vi "Matrix_target.vi"() -> ()   [LabVIEW 2018]
uses:
  <vilib>/Platform/TimedLoop/XDataNode/timing_clust.ctl
  <vilib>/Platform/TimedLoop/XDataNode/nitl_modes.ctl
  <vilib>/Platform/TimedLoop/XDataNode/wakeup.ctl
  <vilib>/rvi/Emulation/niFpgaGetClockAttributes.vi
  <vilib>/rvi/Emulation/niFpgaSctlEmulationGetInTimedLoop.vi
  <vilib>/rvi/Emulation/niFpgaEmulationReportErrorSimple.vi
  <vilib>/rvi/Emulation/niFpgaCriticalErrorInLSC.vi
  <vilib>/rvi/eio/common/nirviEmuTemplateMethod_errors.vi
  <vilib>/rvi/Emulation/niFpgaProcessEmulError.vi
  <vilib>/Platform/TimedLoop/XDataNode/XDataNode.xnode
  <vilib>/eio/EIONode/EIONode.xnode
  <vilib>/Platform/TimedLoop/XDataNode/XDNodeRunTimeDep.lvlib
panel:
  in  "54":i16=53
  in  "36":i16=35
  in  "18":i16=17
  in  "72":i16=53
  in  "71":i16=53
  in  "17":i16=17
  in  "35":i16=35
  in  "53":i16=53
  in  "0_WE divider":i32=10
  in  "10_Rise/Fall divider":i32=3
  in  "75_Stop":i16=57
  out "Data_Array":bool[](array[boolean])
  in  "Send_Request":bool
  in  "DataLow":u64
  out "ACK":bool[](array[boolean])
  in  "/Reset_Bar":bool
  out "Sclk":bool
  in  "DataUp":u64
  in  "100_Sclk_divider":i32=25
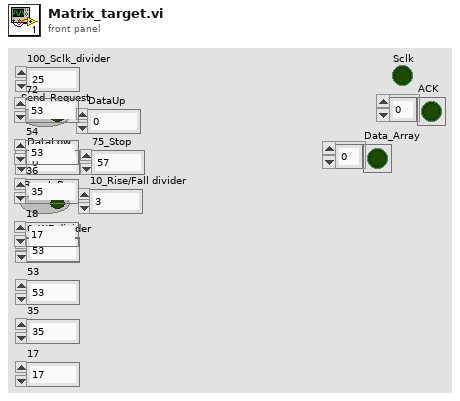
[diagram p1: front panel]
types:
  T1 = typedef "XDNodeRunTimeDep.lvlib/timing_clust.ctl" = cluster{"Expected End [f-1]":u64, "Actual End [f-1]":u64, "Finished Late? [f-1]":bool, "Expected End [i-1]":u64, "Actual End [i-1]":u64, "Finished Late? [i-1]":bool, "Expected Start [i]":u64, "Actual Start [i]":u64, "Expected Start [f]":u64, "Actual Start [f]":u64, "Source Name":string, "Structure Name":string, "Period":i64, "Deadline":i64, "Offset":i64, "Start":i64, "Priority":i32, "Timeout":i32, "Mode":T2, "Wakeup Reason":T3, "Error":errorcluster, "Source Type":string, "Secondary Source Type":string, "Global End Time":u64, "Global Start Time":u64, "Frame Duration":u64, "Iteration Duration":u64, "Assigned CPU":i32, "I/O Scan Engine Mode":u32}
  T2 = typedef "XDNodeRunTimeDep.lvlib/nitl_modes.ctl" = enum32{"No Change", "Process missed periods, maintain original phase", "Discard missed periods, maintain original phase", "Process missed periods, ignore original phase", "Discard missed periods, ignore original phase"}
  T3 = typedef "XDNodeRunTimeDep.lvlib/wakeup.ctl" = enum32{"Normal", "Aborted", "Asynchronous wakeup", "Timing source error", "Timed loop error", "Timeout"}
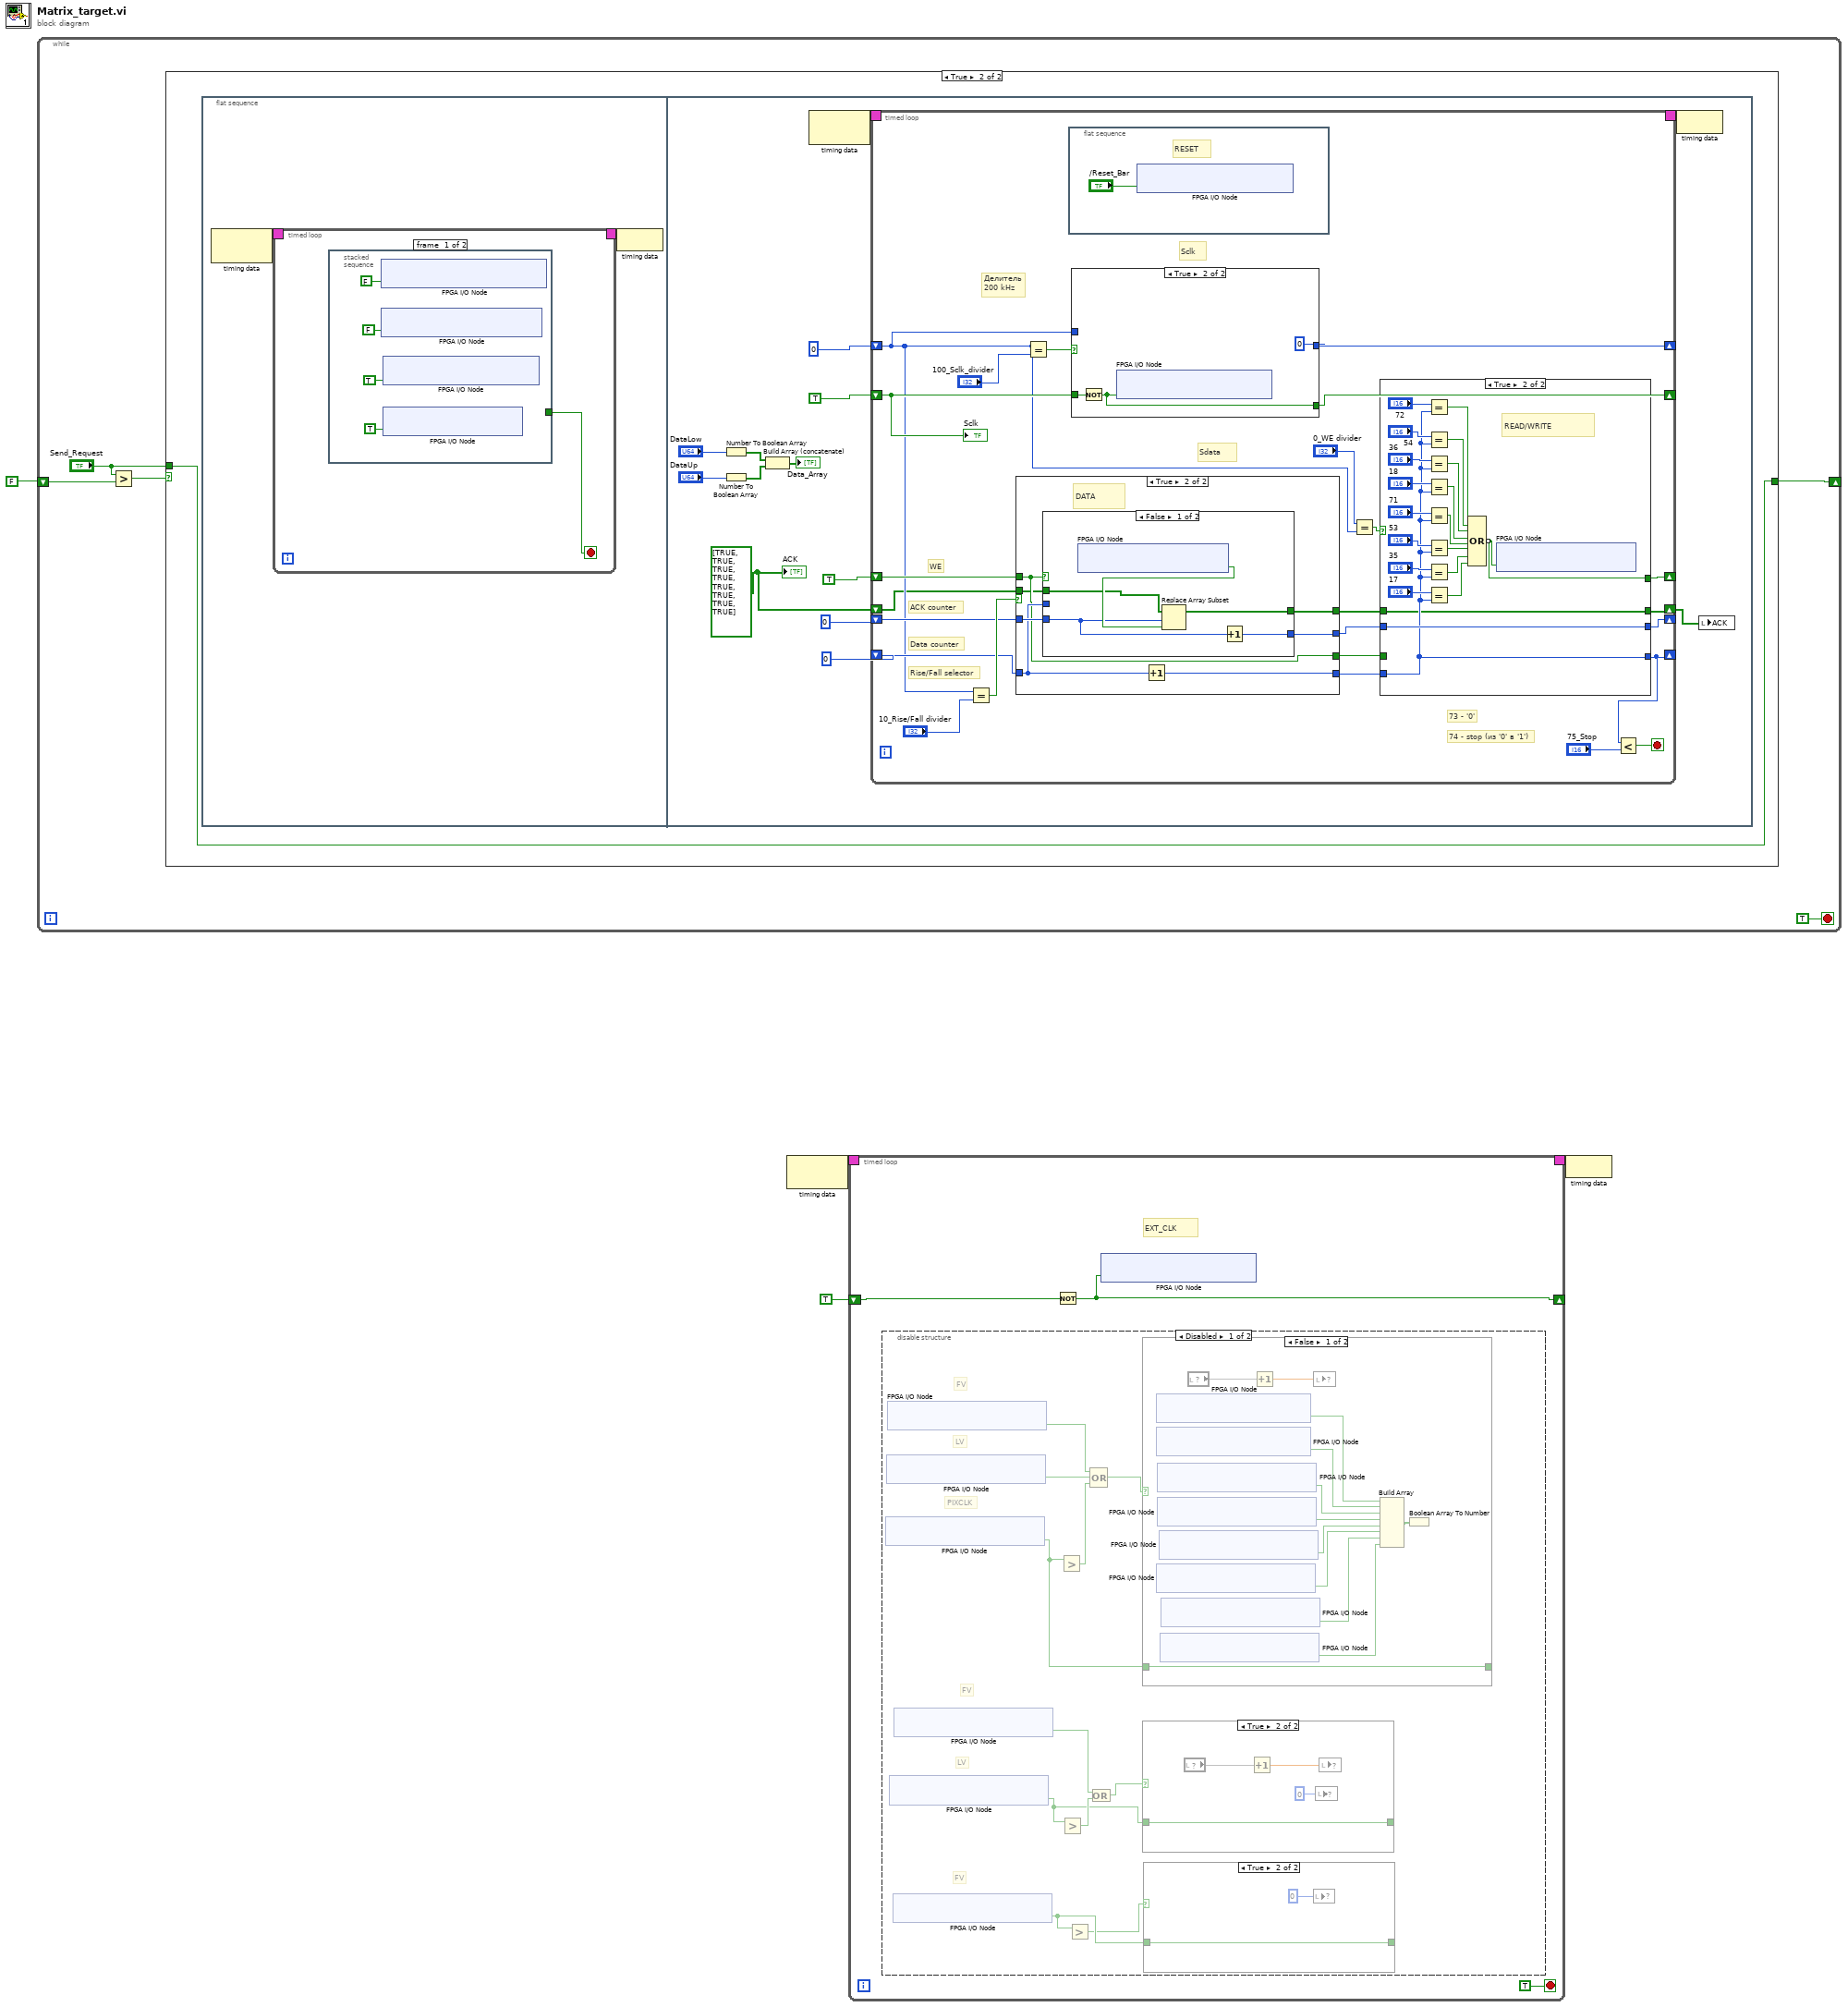
[diagram p0: block diagram]
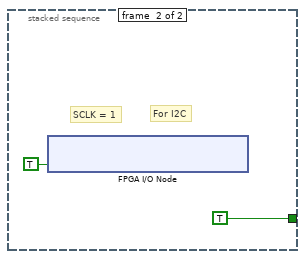
[diagram p7: hidden frame]
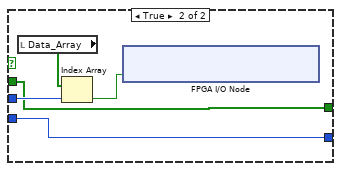
[diagram p10: hidden frame]
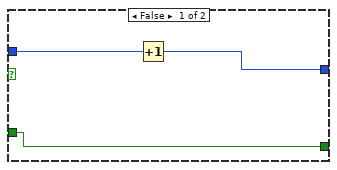
[diagram p11: hidden frame]
diagram:
  n1 = while {
    shift-right: [w8] -> _
    shift-left: FALSE ("Send_Request") -> [w7]
    stop <- TRUE stop-if-true
    n2 = Greater?(x="Send_Request", y=w7) -> (0:w6:bool)
    n3 = case shown="True" w6 {
      tunnel: "Send_Request" -> [w10 w11]
      tunnel: [w10 w11] -> w8
      frame False {
      }
      frame True {
        n4 = flat-sequence {
          frame #0 {
            n5 = node-c288() -> (w13:T1)  [unwired: 1 in]
            n6 = timed-loop {
              timing: w13 -> [_]
              timing-out: [_] -> w12
              stop <- w14 stop-if-true
              n7 = stacked-sequence {
                tunnel: [_ TRUE] -> w14
                frame #0 {
                  n8 = xnode "FPGA I/O Node"("IO Module\\DDCA_DIO16-23_WE"=FALSE ("IO Module\\DDCA_DIO16-23_WE")) -> ()  [unwired: 1 in, 1 out]
                  n9 = xnode "FPGA I/O Node"("IO Module\\DDCA_DIO8-15_WE"=FALSE ("IO Module\\DDCA_DIO8-15_WE")) -> ()  [unwired: 1 in, 1 out]
                  n10 = xnode "FPGA I/O Node"("IO Module\\DDCA_DIO0-7_WE"=TRUE ("IO Module\\DDCA_DIO0-7_WE")) -> ()  [unwired: 1 in, 1 out]
                  n11 = xnode "FPGA I/O Node"("IO Module\\DDCA_PFI_WE"=TRUE ("IO Module\\DDCA_DIO0-7_WE")) -> ()  [unwired: 1 in, 1 out]
                }
                frame #1 {
                  # "For I2C"
                  # "SCLK = 1"
                  n12 = xnode "FPGA I/O Node"("IO Module\\DDCA_DIO6_Write"=TRUE ("IO Module\\DDCA_DIO6_Write")) -> ()  [unwired: 1 in, 1 out]
                }
              }
            }
            n13 = node-c288(w12) -> ()
          }
          frame #1 {
            w25 = bool[] [TRUE, TRUE, TRUE, TRUE, TRUE, TRUE, TRUE, TRUE] ("ACK")
            n14 = Number To Boolean Array(number="DataLow") -> (Boolean array=w32:bool[])
            n15 = Number To Boolean Array(number="DataUp") -> (Boolean array=w31:bool[])
            n16 = Build Array (concatenate)(w32, w31) -> (→"Data_Array":bool[])
            n17 = node-c288() -> (w38:T1)  [unwired: 1 in]
            n18 = timed-loop {
              timing: w38 -> [_]
              timing-out: [_] -> w37
              shift-right: [w61] -> _
              shift-left: 0 -> [w50]
              shift-right: [w60] -> _
              shift-left: TRUE ("IO Module\\DDCA_DIO0_Write") -> [w57]
              shift-right: [w47] -> _
              shift-left: i16 0 -> [w55]
              shift-right: [w45] -> _
              shift-left: i16 0 -> [w54]
              shift-right: [w44] -> _
              shift-left: TRUE -> [w53]
              shift-right: [w40] -> w26
              shift-left: w25 -> [w39]
              stop <- w42 stop-if-true
              # "Rise/Fall selector"
              # "WE"
              # "Data counter"
              # "ACK counter"
              # "74 - stop (из '0' в '1')"
              # "73 - '0'"
              # "Sdata"
              # "Sclk"
              # "Делитель\n200 kHz"
              n19 = Equal?(x=w50, y="10_Rise/Fall divider") -> (x = y?=w56:bool)
              n20 = case shown="True" w56 {
                tunnel: [w89 w93] -> w48
                tunnel: w55 -> [w89 w95]
                tunnel: w54 -> [w90 w97]
                tunnel: [w90 w96] -> w46
                tunnel: w53 -> [w88 w94]
                tunnel: [w88 w94] -> w43
                tunnel: [w87 w92] -> w41
                tunnel: w39 -> [w87 w91]
                frame False {
                }
                frame True {
                  # "DATA"
                  n21 = case shown="False" w94 {
                    tunnel: w97 -> [w101 w107]
                    tunnel: [w100 w107] -> w96
                    tunnel: w95 -> [_ w106]
                    tunnel: [w99 w103] -> w92
                    tunnel: w91 -> [w98 w103]
                    frame False {
                      n22 = xnode "FPGA I/O Node"() -> ("IO Module\\DDCA_PFI1_Read"=w102:bool)  [unwired: 1 in, 1 out]
                      n23 = Replace Array Subset(array=w98, new element=w102, index=w101) -> (w99:bool[])
                      n24 = Increment(x=w101) -> (x+1=w100:i16)
                    }
                    frame True {
                      n25 = local read "Data_Array"() -> (w105:bool[])
                      n26 = Index Array(array=w105, index=w106) -> (element=w104:bool)
                      n27 = xnode "FPGA I/O Node"("IO Module\\DDCA_PFI1_Write"=w104) -> ()  [unwired: 1 in, 1 out]
                    }
                  }
                  n28 = Increment(x=w95) -> (x+1=w93:i16)
                }
              }
              n29 = Equal?(x=w50, y="100_Sclk_divider") -> (x = y?=w62:bool)
              n30 = flat-sequence {
                frame #0 {
                  # "RESET"
                  n31 = xnode "FPGA I/O Node"("IO Module\\DDCA_DIO5_Write"="/Reset_Bar") -> ()  [unwired: 1 in, 1 out]
                }
              }
              n32 = case shown="True" w62 {
                tunnel: [w110 0] -> w61
                tunnel: w50 -> [w111 _]
                tunnel: w57 -> [w109 w113]
                tunnel: [w109 w112] -> w60
                frame False {
                  n33 = Increment(x=w111) -> (x+1=w110:i32)
                }
                frame True {
                  n34 = Not(x=w113) -> (.not. x?=w112:bool)
                  n35 = xnode "FPGA I/O Node"("IO Module\\DDCA_DIO6_Write"=w112) -> ()  [unwired: 1 in, 1 out]
                }
              }
              n36 = Equal?(x="0_WE divider", y=w50) -> (x = y?=w49:bool)
              n37 = case shown="True" w49 {
                tunnel: w48 -> [w65 w72]
                tunnel: [w65 w72] -> w47
                tunnel: [w66 w78] -> w45
                tunnel: w46 -> [w66 w78]
                tunnel: [w64 w77] -> w44
                tunnel: w43 -> [w64 _]
                tunnel: w41 -> [w63 w67]
                tunnel: [w63 w67] -> w40
                frame False {
                }
                frame True {
                  # "READ/WRITE"
                  n38 = Equal?(x="72", y=w72) -> (x = y?=w71:bool)
                  n39 = Equal?(x="54", y=w72) -> (x = y?=w68:bool)
                  n40 = Equal?(x="36", y=w72) -> (x = y?=w70:bool)
                  n41 = Equal?(x="18", y=w72) -> (x = y?=w69:bool)
                  n42 = Equal?(x="71", y=w72) -> (x = y?=w79:bool)
                  n43 = Equal?(x="53", y=w72) -> (x = y?=w82:bool)
                  n44 = Equal?(x="35", y=w72) -> (x = y?=w84:bool)
                  n45 = Equal?(x="17", y=w72) -> (x = y?=w86:bool)
                  n46 = Compound Arithmetic op=OR(w71, w68, w70, w69, w79, w82, w84, w86) -> (invert w77:bool)
                  n47 = xnode "FPGA I/O Node"("IO Module\\DDCA_PFI_WE"=w77) -> ()  [unwired: 1 in, 1 out]
                }
              }
              n48 = Less?(x=w47, y="75_Stop") -> (x < y?=w42:bool)
              "Sclk" <- w57
            }
            n49 = node-c288(w37) -> ()
            n50 = local write "ACK"(w26) -> ()
            "ACK" <- w25
          }
        }
      }
    }
  }
  n51 = node-c288() -> (w3:T1)  [unwired: 1 in]
  n52 = timed-loop {
    timing: w3 -> [_]
    timing-out: [_] -> w2
    shift-right: [w119] -> _
    shift-left: TRUE -> [w120]
    stop <- TRUE stop-if-true
    # "EXT_CLK"
    n53 = disable-structure shown="Disabled" {
      frame Disabled {
        # "FV"
        # "LV"
        # "FV"
        # "PIXCLK"
        # "LV"
        # "FV"
        n54 = xnode "FPGA I/O Node"() -> ("IO Module\\DDCA_DIO17_Read"=w126:bool)  [unwired: 1 in, 1 out]
        n55 = xnode "FPGA I/O Node"() -> ("IO Module\\DDCA_DIO22_Read"=w131:bool)  [unwired: 1 in, 1 out]
        n56 = xnode "FPGA I/O Node"() -> ("IO Module\\DDCA_DIO23_Read"=w130:bool)  [unwired: 1 in, 1 out]
        n57 = xnode "FPGA I/O Node"() -> ("IO Module\\DDCA_DIO22_Read"=w124:bool)  [unwired: 1 in, 1 out]
        n58 = xnode "FPGA I/O Node"() -> ("IO Module\\DDCA_DIO23_Read"=w123:bool)  [unwired: 1 in, 1 out]
        n59 = xnode "FPGA I/O Node"() -> ("IO Module\\DDCA_DIO23_Read"=w128:bool)  [unwired: 1 in, 1 out]
        n60 = Greater?(x=w126) -> (0:w132:bool)  [unwired: 1 in]
        n61 = Greater?(x=w124) -> (0:w125:bool)  [unwired: 1 in]
        n62 = Greater?(x=w123) -> (0:w122:bool)  [unwired: 1 in]
        n63 = Compound Arithmetic op=OR(w130, w131, w132) -> (w129:bool)
        n64 = Compound Arithmetic op=OR(w128, w125) -> (w127:bool)
        n65 = case shown="False" w129 {
          tunnel: [w152 w153] -> _
          tunnel: w126 -> [w152 w153]
          frame False {
            n66 = xnode "FPGA I/O Node"() -> ("IO Module\\DDCA_DIO8_Read"=w149:bool)  [unwired: 1 in, 1 out]
            n67 = xnode "FPGA I/O Node"() -> ("IO Module\\DDCA_DIO9_Read"=w148:bool)  [unwired: 1 in, 1 out]
            n68 = xnode "FPGA I/O Node"() -> ("IO Module\\DDCA_DIO13_Read"=w144:bool)  [unwired: 1 in, 1 out]
            n69 = xnode "FPGA I/O Node"() -> ("IO Module\\DDCA_DIO10_Read"=w147:bool)  [unwired: 1 in, 1 out]
            n70 = xnode "FPGA I/O Node"() -> ("IO Module\\DDCA_DIO11_Read"=w146:bool)  [unwired: 1 in, 1 out]
            n71 = xnode "FPGA I/O Node"() -> ("IO Module\\DDCA_DIO12_Read"=w145:bool)  [unwired: 1 in, 1 out]
            n72 = xnode "FPGA I/O Node"() -> ("IO Module\\DDCA_DIO13_Read"=w142:bool)  [unwired: 1 in, 1 out]
            n73 = xnode "FPGA I/O Node"() -> ("IO Module\\DDCA_DIO13_Read"=w143:bool)  [unwired: 1 in, 1 out]
            n74 = local read item#-1() -> (w151)
            n75 = Increment(x=w151) -> (x+1=w150:dbl)
            n76 = local write item#-1(w150) -> ()
            n77 = Build Array(w149, w148, w147, w146, w145, w144, w143, w142) -> (w141:bool[])
            n78 = Boolean Array To Number(Boolean array=w141) -> ()  [unwired: 1 out]
          }
          frame True {
          }
        }
        n79 = case shown="True" w127 {
          tunnel: w124 -> [w136 w140]
          tunnel: [w136 w140] -> _
          frame False {
          }
          frame True {
            n80 = local read item#-1() -> (w139)
            n81 = Increment(x=w139) -> (x+1=w138:dbl)
            n82 = local write item#-1(i16 0 ("Pix")) -> ()
            n83 = local write item#-1(w138) -> ()
          }
        }
        n84 = case shown="True" w122 {
          tunnel: w123 -> [w133 w135]
          tunnel: [w133 w135] -> _
          frame False {
          }
          frame True {
            n85 = local write item#-1(i16 0 ("Lines")) -> ()
          }
        }
      }
      frame Enabled {
      }
    }
    n86 = Not(x=w120) -> (.not. x?=w119:bool)
    n87 = xnode "FPGA I/O Node"("IO Module\\DDCA_DIO7_Write"=w119) -> ()  [unwired: 1 in, 1 out]
  }
  n88 = node-c288(w2) -> ()
